vi "TDTtester.vi"   [LabVIEW 2014]
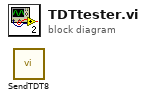
[diagram p0: block diagram]
diagram:
  n1 = call "SendTDT8.vi"() -> ()  [unwired: 5 in]
